vi "host.vi"() -> ()   [LabVIEW 2020]
uses:
  <vilib>/FPGAPlugInAG/cRIO-9035/niLvFpga_Open_cRIO-9035.vi
  <vilib>/rvi/interface/common/dynamic/niFpgaDynamicAddResources.vi
  <vilib>/Utility/error.llb/Error Cluster From Error Code.vi
  <vilib>/rvi/errors/niLvFpgaAdjustHostInterfaceError.vi
  <vilib>/FPGAPlugInAG/Dynamic/niLvFpga_Run_Dynamic.vi
  <vilib>/FPGAPlugInAG/Dynamic/niLvFpga_Close_Dynamic.vi
  <vilib>/rvi/interface/nirviOpenFPGA/nirviOpenFPGA.xnode
  FPGA Bitfiles/4.5.7_FPGATarget_target_Djorh8G557E.lvbitx
  target.vi
  <vilib>/rvi/interface/nirviMethod/nirviMethod.xnode
  <vilib>/rvi/interface/nirviCloseFPGA/nirviCloseFPGA.xnode
  <vilib>/rvi/errors/niLvFpgaMergeErrorWithErrorCode.vi
  <vilib>/FPGAPlugInAG/Dynamic/niLvFpga_ReadFifo_Dynamic.vi
  <vilib>/FPGAPlugInAG/Dynamic/niLvFpga_WriteFifo_Dynamic.vi
panel:
  out "Tick end for total":fxp<+/-,32,16>[](array[numeric])
  out "Tick start for total":fxp<+/-,32,16>[](array[numeric])
  out "start tick":fxp<+/-,32,16>[](array[numeric])
  out "Data IN":fxp<+/-,32,16>[](array[numeric])
  out "MLP forward pass":fxp<+/-,32,16>[](array[numeric])
  out "data manipulation":fxp<+/-,32,16>[](array[numeric])
  out "Subsampling":fxp<+/-,32,16>[](array[numeric])
  out "Attention layer and\n backpropagation":fxp<+/-,32,16>[](array[numeric])
  out "end tick":fxp<+/-,32,16>[](array[numeric])
  out "data output":dbl[][](graph)
  out "MLP 1 size(s)":i32
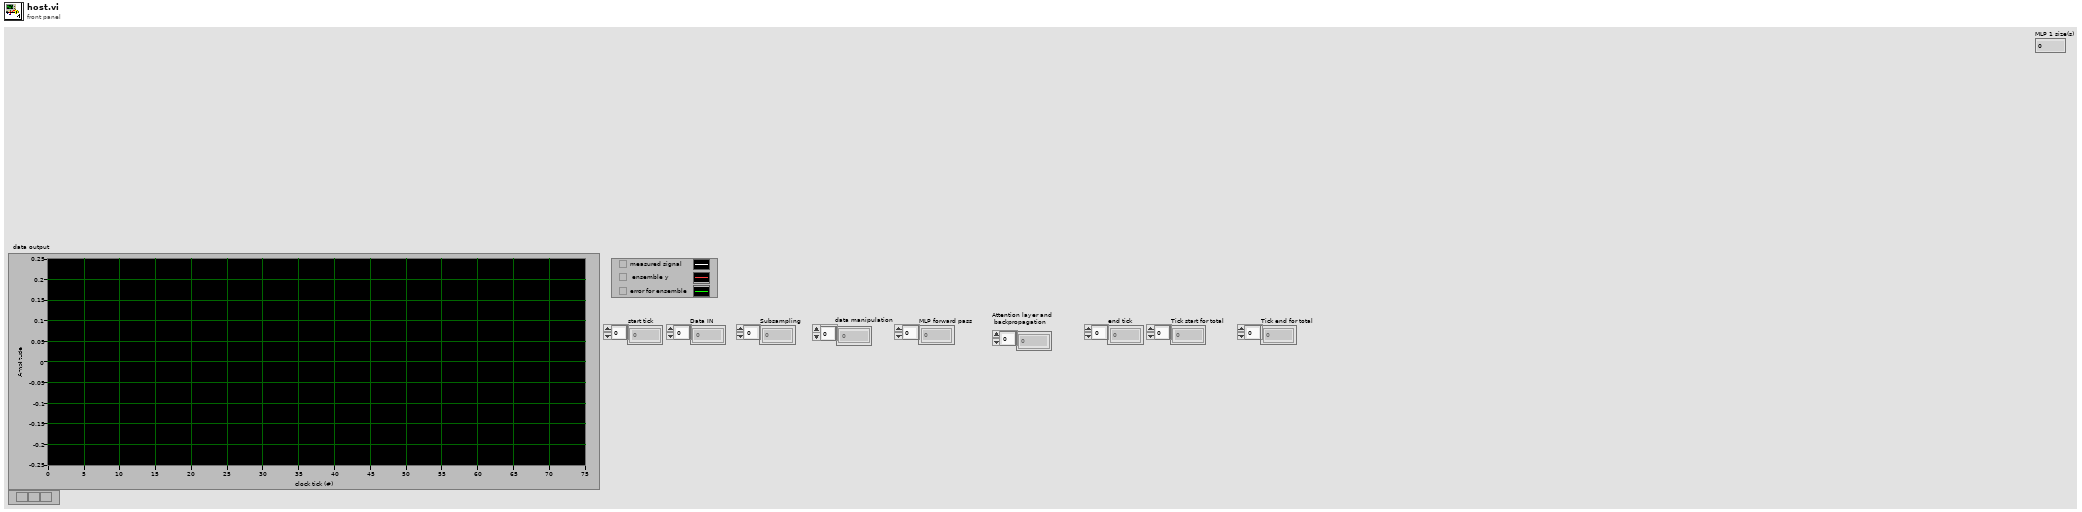
[diagram p1: front panel]
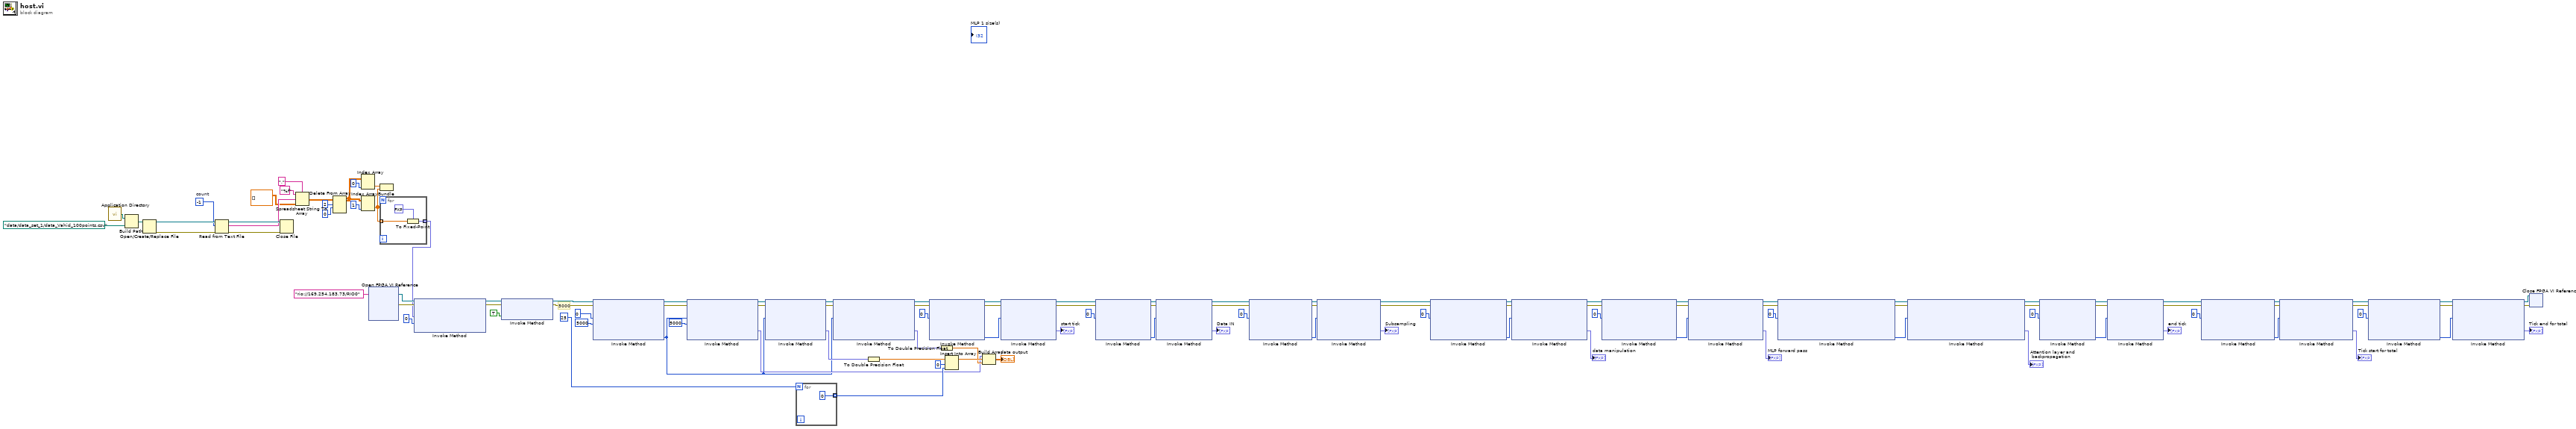
[diagram p0: block diagram]
diagram:
  w96 = -1  # count
  # "5000"
  n1 = call <vilib>:"Application Directory.vi"() -> ("Application Directory"=w100:path)
  n2 = Build Path(base path=w100, name or relative path=path "data/data_set_1/data_Vahid_100points.csv" ("default name")) -> (appended path=w99:path)
  n3 = Open/Create/Replace File(file path (use dialog)=w99) -> (refnum out=w104:refnum<file>, error out=w105:errorcluster)  [unwired: 5 in, 1 out]
  n4 = Read from Text File(file (use dialog)=w104, count=w96, error in=w105) -> (refnum out=w103:refnum<file>, text=w101:string, error out=w102:errorcluster)  [unwired: 1 in, 1 out]
  n5 = Close File(refnum=w103, error in=w102) -> ()  [unwired: 2 out]
  n6 = Spreadsheet String To Array(delimiter (Tab)=",", format string="%f", spreadsheet string=w101, array type (2D Dbl)=dbl[][] []) -> (array=w93:dbl[][])
  n7 = Delete From Array(array=w93, length=2, index (row)=0) -> (array with subset deleted=w87:dbl[][])  [unwired: 1 in, 1 out]
  n8 = Index Array(array=w87, index (col)=0 ("disabled index (col)")) -> (element=w81:dbl[])  [unwired: 1 in]
  n9 = Index Array(array=w87, index (col)=1 ("disabled index (col)")) -> (element=w89:dbl[])  [unwired: 1 in]
  n10 = xnode "Open FPGA VI Reference"("resource name"=tag "rio://169.254.183.73/RIO0") -> ("FPGA VI Reference Out"=w112:refnum<k20>, "error out"=w111:errorcluster)  [unwired: 1 in]
  n11 = Bundle("array type (2D Dbl)"=w81, "array type (2D Dbl)"=w89) -> ()  [unwired: 1 in, 1 out]
  n12 = for {
    tunnel: [w117] -> w83 mode=indexing
    tunnel: w89 -> [w116] mode=indexing
    n13 = To Fixed-Point(fixed-point type=fxp<+/-,32,16> 0.0 ("f"), number=w116) -> (fixed-point=w117:fxp<+/-,32,16>)
  }
  n14 = xnode "Invoke Method"("FPGA VI Reference In"=w112, "error in"=w111, "Data"=w83, "Timeout (ms)"=0) -> ("FPGA VI Reference Out"=w110:refnum<k20>, "error out"=w109:errorcluster)  [unwired: 1 out]
  n15 = xnode "Invoke Method"("FPGA VI Reference In"=w110, "error in"=w109, "Wait Until Done (F)"=TRUE) -> ("FPGA VI Reference Out"=w114:refnum<k20>, "error out"=w113:errorcluster)
  n16 = xnode "Invoke Method"("FPGA VI Reference In"=w114, "error in"=w113, "Number of Elements"=u32 0, "Timeout (ms)"=5000) -> ("FPGA VI Reference Out"=w108:refnum<k20>, "error out"=w107:errorcluster, "Elements Remaining"=w66:u32)  [unwired: 1 out]
  n17 = xnode "Invoke Method"("FPGA VI Reference In"=w108, "error in"=w107, "Number of Elements"=w66, "Timeout (ms)"=5000) -> ("FPGA VI Reference Out"=w80:refnum<k20>, "error out"=w79:errorcluster, "Data"=w68:fxp<+/-,32,16>[])  [unwired: 1 out]
  n18 = xnode "Invoke Method"("FPGA VI Reference In"=w80, "error in"=w79, "Number of Elements"=w66) -> ("FPGA VI Reference Out"=w78:refnum<k20>, "error out"=w77:errorcluster, "Data"=w70:fxp<+/-,32,16>[])  [unwired: 1 in, 1 out]
  n19 = for {
    N: 25 -> [_]
    tunnel: [0] -> w74 mode=indexing
  }
  n20 = xnode "Invoke Method"("FPGA VI Reference In"=w78, "error in"=w77, "Number of Elements"=w66) -> ("FPGA VI Reference Out"=w27:refnum<k20>, "error out"=w26:errorcluster, "Data"=w69:fxp<+/-,32,16>[])  [unwired: 1 in, 1 out]
  n21 = To Double Precision Float(number=w70) -> (double precision float=w67:dbl[])
  n22 = xnode "Invoke Method"("FPGA VI Reference In"=w27, "error in"=w26, "Number of Elements"=u32 0) -> ("FPGA VI Reference Out"=w52:refnum<k20>, "error out"=w51:errorcluster, "Elements Remaining"=w50:u32)  [unwired: 1 in, 1 out]
  n23 = To Double Precision Float(number=w69) -> (double precision float=w71:dbl[])
  n24 = Insert Into Array(array=w67, index=0, new element=w74) -> (w72:dbl[])
  n25 = Build Array(w68, w72, w71) -> (→"data output":dbl[][])
  n26 = xnode "Invoke Method"("FPGA VI Reference In"=w52, "error in"=w51, "Number of Elements"=w50) -> ("FPGA VI Reference Out"=w25:refnum<k20>, "error out"=w24:errorcluster, "Data"=→"start tick":fxp<+/-,32,16>[])  [unwired: 1 in, 1 out]
  n27 = xnode "Invoke Method"("FPGA VI Reference In"=w25, "error in"=w24, "Number of Elements"=u32 0) -> ("FPGA VI Reference Out"=w40:refnum<k20>, "error out"=w39:errorcluster, "Elements Remaining"=w38:u32)  [unwired: 1 in, 1 out]
  n28 = xnode "Invoke Method"("FPGA VI Reference In"=w40, "error in"=w39, "Number of Elements"=w38) -> ("FPGA VI Reference Out"=w29:refnum<k20>, "error out"=w28:errorcluster, "Data"=→"Data IN":fxp<+/-,32,16>[])  [unwired: 1 in, 1 out]
  n29 = xnode "Invoke Method"("FPGA VI Reference In"=w29, "error in"=w28, "Number of Elements"=u32 0) -> ("FPGA VI Reference Out"=w48:refnum<k20>, "error out"=w47:errorcluster, "Elements Remaining"=w46:u32)  [unwired: 1 in, 1 out]
  n30 = xnode "Invoke Method"("FPGA VI Reference In"=w48, "error in"=w47, "Number of Elements"=w46) -> ("FPGA VI Reference Out"=w31:refnum<k20>, "error out"=w30:errorcluster, "Data"=→"Subsampling":fxp<+/-,32,16>[])  [unwired: 1 in, 1 out]
  n31 = xnode "Invoke Method"("FPGA VI Reference In"=w31, "error in"=w30, "Number of Elements"=u32 0) -> ("FPGA VI Reference Out"=w44:refnum<k20>, "error out"=w43:errorcluster, "Elements Remaining"=w42:u32)  [unwired: 1 in, 1 out]
  n32 = xnode "Invoke Method"("FPGA VI Reference In"=w44, "error in"=w43, "Number of Elements"=w42) -> ("FPGA VI Reference Out"=w33:refnum<k20>, "error out"=w32:errorcluster, "Data"=→"data manipulation":fxp<+/-,32,16>[])  [unwired: 1 in, 1 out]
  n33 = xnode "Invoke Method"("FPGA VI Reference In"=w33, "error in"=w32, "Number of Elements"=u32 0) -> ("FPGA VI Reference Out"=w56:refnum<k20>, "error out"=w55:errorcluster, "Elements Remaining"=w54:u32)  [unwired: 1 in, 1 out]
  n34 = xnode "Invoke Method"("FPGA VI Reference In"=w56, "error in"=w55, "Number of Elements"=w54) -> ("FPGA VI Reference Out"=w35:refnum<k20>, "error out"=w34:errorcluster, "Data"=→"MLP forward pass":fxp<+/-,32,16>[])  [unwired: 1 in, 1 out]
  n35 = xnode "Invoke Method"("FPGA VI Reference In"=w35, "error in"=w34, "Number of Elements"=u32 0) -> ("FPGA VI Reference Out"=w60:refnum<k20>, "error out"=w59:errorcluster, "Elements Remaining"=w58:u32)  [unwired: 1 in, 1 out]
  n36 = xnode "Invoke Method"("FPGA VI Reference In"=w60, "error in"=w59, "Number of Elements"=w58) -> ("FPGA VI Reference Out"=w37:refnum<k20>, "error out"=w36:errorcluster, "Data"=→"Attention layer and\n backpropagation":fxp<+/-,32,16>[])  [unwired: 1 in, 1 out]
  n37 = xnode "Invoke Method"("FPGA VI Reference In"=w37, "error in"=w36, "Number of Elements"=u32 0) -> ("FPGA VI Reference Out"=w64:refnum<k20>, "error out"=w63:errorcluster, "Elements Remaining"=w62:u32)  [unwired: 1 in, 1 out]
  n38 = xnode "Invoke Method"("FPGA VI Reference In"=w64, "error in"=w63, "Number of Elements"=w62) -> ("FPGA VI Reference Out"=w1:refnum<k20>, "error out"=w11:errorcluster, "Data"=→"end tick":fxp<+/-,32,16>[])  [unwired: 1 in, 1 out]
  n39 = xnode "Invoke Method"("FPGA VI Reference In"=w1, "error in"=w11, "Number of Elements"=u32 0) -> ("FPGA VI Reference Out"=w17:refnum<k20>, "error out"=w16:errorcluster, "Elements Remaining"=w15:u32)  [unwired: 1 in, 1 out]
  n40 = xnode "Invoke Method"("FPGA VI Reference In"=w17, "error in"=w16, "Number of Elements"=w15) -> ("FPGA VI Reference Out"=w10:refnum<k20>, "error out"=w9:errorcluster, "Data"=→"Tick start for total":fxp<+/-,32,16>[])  [unwired: 1 in, 1 out]
  n41 = xnode "Invoke Method"("FPGA VI Reference In"=w10, "error in"=w9, "Number of Elements"=u32 0) -> ("FPGA VI Reference Out"=w14:refnum<k20>, "error out"=w13:errorcluster, "Elements Remaining"=w12:u32)  [unwired: 1 in, 1 out]
  n42 = xnode "Invoke Method"("FPGA VI Reference In"=w14, "error in"=w13, "Number of Elements"=w12) -> ("FPGA VI Reference Out"=w8:refnum<k20>, "error out"=w7:errorcluster, "Data"=→"Tick end for total":fxp<+/-,32,16>[])  [unwired: 1 in, 1 out]
  n43 = xnode "Close FPGA VI Reference"("FPGA VI Reference In"=w8, "error in"=w7) -> ()  [unwired: 1 out]
